vi "CRef Variant Core.vi"(7 "Type":T1, 9 "Operation":enum16{"Create", "Read", "Write", "Release"}(ring), 10 "Index":u16, 11 "Item":bool) -> (2 "Index":u16, 3 "Item":bool)   [LabVIEW 2012, in "CRef.lvlib"]
uses:
  CRef.lvlib
  Master Types.ctl
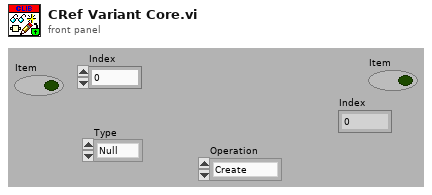
[diagram p1: front panel]
types:
  T1 = typedef "CRef.lvlib/Master Types.ctl" = enum8{"Null", "Boolean", "U8", "I8", "U16", "I16", "U32", "I32", "U64", "I64", "Single", "Double", "Extended", "CSG", "CDB", "CXT", "Boolean(Def)", "U8(Def)", "I8(Def)", "U16(Def)", "I16(Def)", "U32(Def)", "I32(Def)", "Reserved Def", "Reserved Def1", "Single(Def)", "Double(Def)", "Reserved Def2", "Reserved Def3", "Reserved Def4", "Reserved Def5", "Unsigned(Def)", "Signed(Def)", "Real(Def)", "Reserved Def6", "Numeric(Def)", "String"}
  T2 = enum8{"1-bit", "8-bit", "16-bit", "32-bit", "64-bit", "Variant"}
  T3 = typedef "CRef.lvlib/Variant CReference.ctl" = cluster{"Generic CRef Address":u16, "Type":u8}
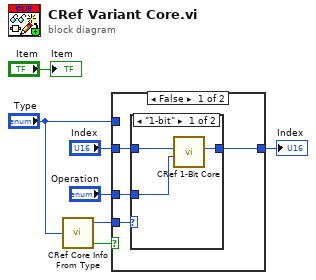
[diagram p0: block diagram]
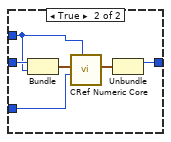
[diagram p3: hidden frame]
diagram:
  n1 = call "CRef Core Info From Type.vi"("Type"="Type") -> ("Numeric?"=w2:bool, "Specific Core"=w3:T2)  [unwired: 2 in, 1 out]
  n2 = case shown="False" w2 {
    tunnel: "Index" -> [w11 w20]
    tunnel: "Operation" -> [w10 w15]
    tunnel: [w9 w17] -> w4
    tunnel: w3 -> [w8 _]
    tunnel: "Type" -> [_ w16]
    frame False {
      n3 = case shown="\"1-bit\"" w8 {
        tunnel: w11 -> [w14 _]
        tunnel: w10 -> [w13 _]
        tunnel: [w12 _] -> w9
        frame "1-bit" {
          n4 = call "CRef 1-Bit Core.vi"("Operation"=w13, "Index"=w14) -> ("Index"=w12:u16)  [unwired: 8 in, 1 out]
        }
        frame Default {
        }
      }
    }
    frame True {
      n5 = Bundle("Index"=w20, "Type"=w16) -> (w19:cluster{"Index":u16, "Type":T1})  [unwired: 1 in]
      n6 = call "CRef Numeric Core.vi"("Operator Type"=w16, "Operation"=w15, "Address"=w19) -> ("Address"=w18:T3)  [unwired: 7 in, 1 out]
      n7 = Unbundle(w18) -> ("Generic CRef Address"=w17:u16)  [unwired: 1 out]
    }
  }
  "Index" <- w4
  "Item" <- "Item"
